vi "subvi_crenelation_reader.vi"(8 "Current Angles":cluster{"Analyser 1":i32, "Analyser 2":i32}, 9 "file (use dialog) 2":path, 10 "Directions":cluster{"Analyser 1":bool, "Analyser 2":bool}, 11 "Analysers Moving?":T1) -> (0 "New Current Angles":cluster{"Analyser 1":i32, "Analyser 2":i32}, 1 "Crenelation \nInterrupts":bool[](array[boolean]) caption="Crenelation Indicators", 3 "Analysers Moving? Output":T1)   [LabVIEW 2014]
doc: "Reads crenelation interrupt (Port 1.1 for analyser 1 and Port 1.5 for analyser 2) states and increments the current angle by 5 degrees if an interrupt fires and appends the new angle to a file specified."
uses:
  Bool Crossing/typedef_twice_bool_crossing.ctl
panel:
  # "INPUTS"
  # "OUTPUTS"
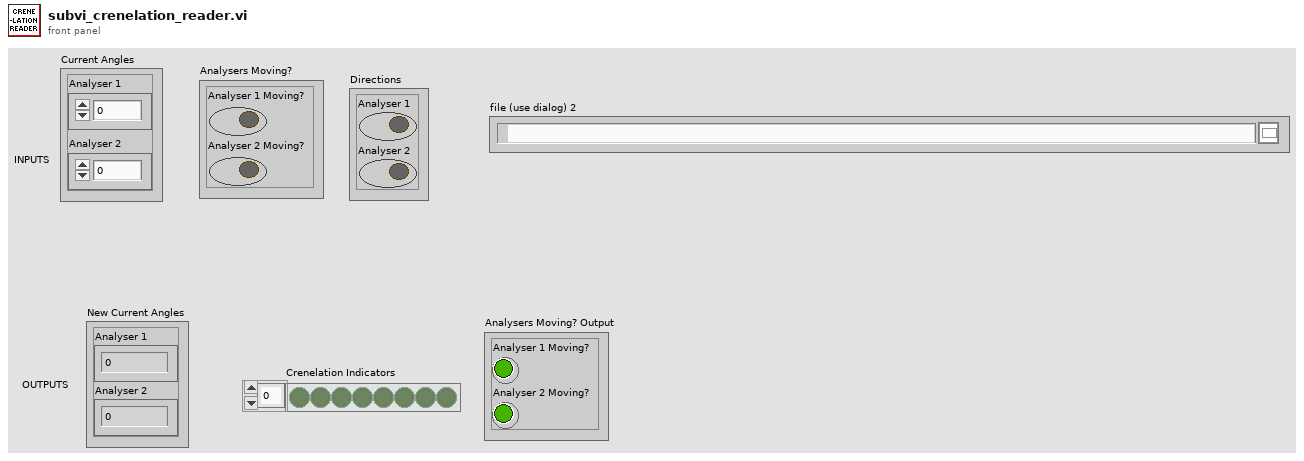
[diagram p1: front panel]
types:
  T1 = cluster{"Analyser 1 Moving?":bool, "Analyser 2 Moving?":bool}
  T2 = typedef "typedef_twice_bool_crossing.ctl" = enum16{"F->T->F", "T->F->T", "Initialise"}
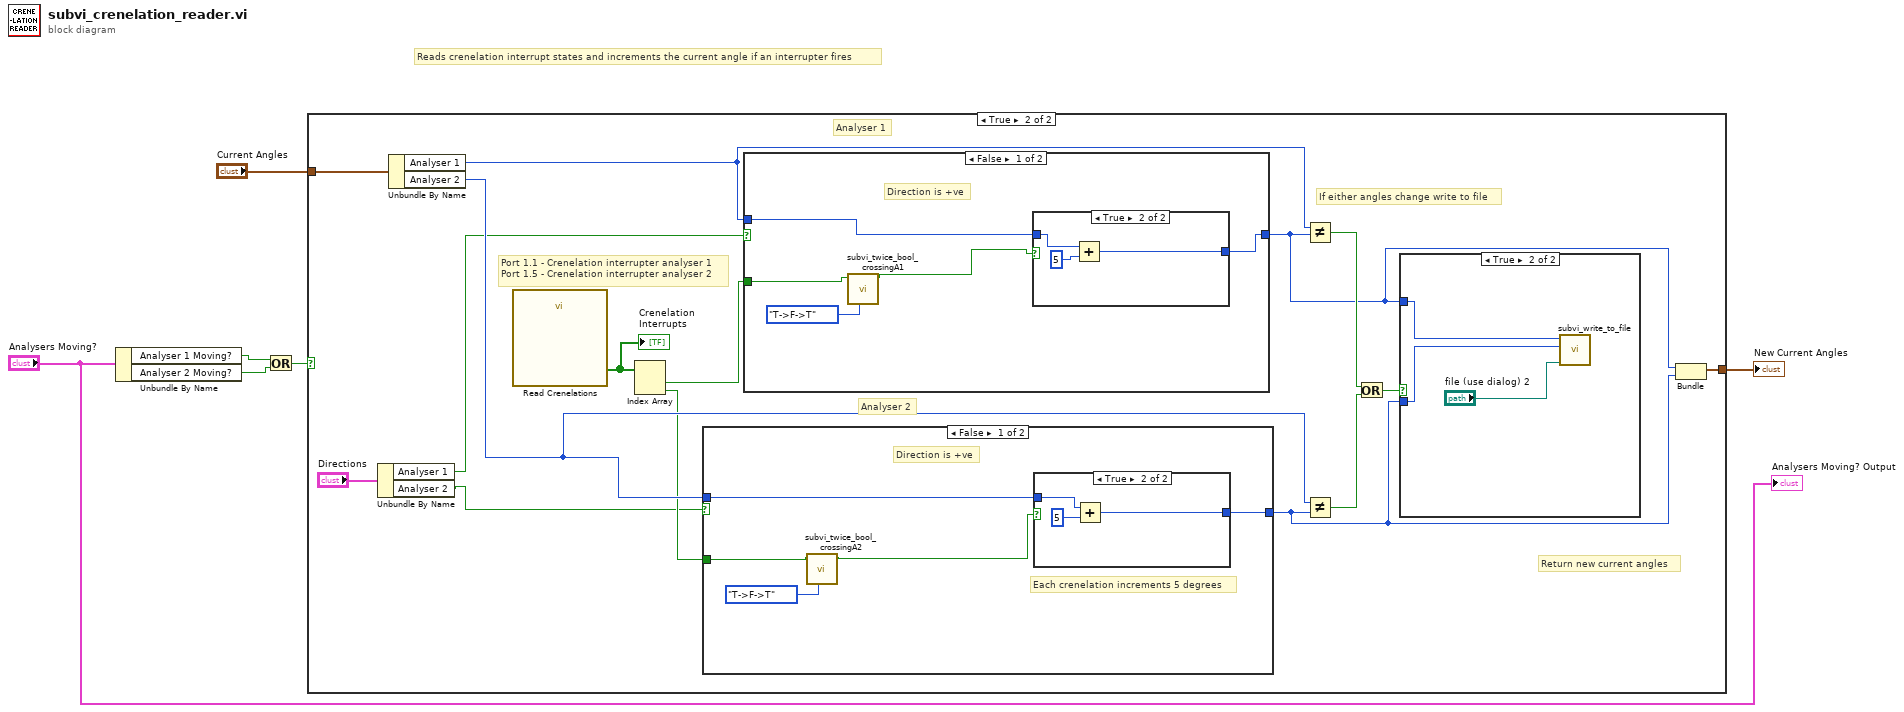
[diagram p0: block diagram]
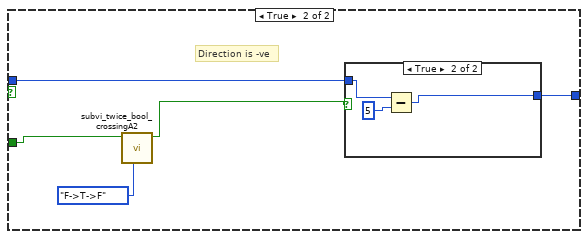
[diagram p4: hidden frame]
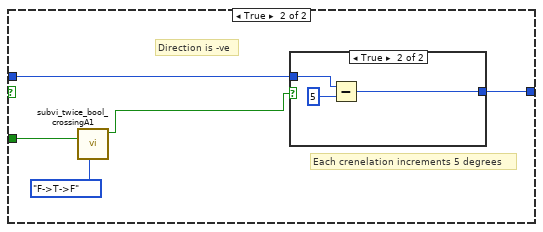
[diagram p8: hidden frame]
diagram:
  # "Reads crenelation interrupt states and increments the current angle if an interrupter fires"
  n1 = Unbundle By Name("Analysers Moving?") -> ("Analyser 1 Moving?"=w5:bool, "Analyser 2 Moving?"=w4:bool)
  n2 = Or(x=w5, y=w4) -> (x .or. y?=w3:bool)
  n3 = case shown="True" w3 {
    tunnel: [w7 w8] -> w2
    tunnel: "Current Angles" -> [w7 w9]
    frame False {
    }
    frame True {
      # "Analyser 2"
      # "Return new current angles"
      # "If either angles change write to file"
      # "Analyser 1"
      # "Port 1.1 - Crenelation interrupter analyser 1\nPort 1.5 - Crenelation interrupter analyser 2"
      n4 = Unbundle By Name("Directions") -> ("Analyser 1"=w12:bool, "Analyser 2"=w11:bool)
      n5 = Unbundle By Name(w9) -> ("Analyser 1"=w19:i32, "Analyser 2"=w18:i32)
      n6 = call "Read Crenelations"() -> ("data"=w15:bool[])  [unwired: 17 in, 2 out]
      "Crenelation \nInterrupts" <- w15
      n7 = Index Array(array=w15) -> (element #1=w14:bool, element #2=w13:bool)  [unwired: 2 in]
      n8 = case shown="False" w11 {
        tunnel: w13 -> [w25 w34]
        tunnel: w18 -> [w27 w36]
        tunnel: [w26 w35] -> w16
        frame False {
          # "Each crenelation increments 5 degrees"
          # "Direction is +ve"
          n9 = call "subvi_twice_bool_crossingA2.vi"("Action"=typedef_twice_bool_crossing."T->F->T", "Input Bool"=w25) -> ("Action Met?"=w24:bool)  [unwired: 8 in, 1 out]
          n10 = case shown="True" w24 {
            tunnel: w27 -> [w28 w31]
            tunnel: [w28 w29] -> w26
            frame False {
            }
            frame True {
              n11 = Add(x=w31, y=5) -> (x+y=w29:i32)
            }
          }
        }
        frame True {
          # "Direction is -ve"
          n12 = call "subvi_twice_bool_crossingA2.vi"("Action"=typedef_twice_bool_crossing."F->T->F", "Input Bool"=w34) -> ("Action Met?"=w33:bool)  [unwired: 8 in, 1 out]
          n13 = case shown="True" w33 {
            tunnel: w36 -> [w37 w40]
            tunnel: [w37 w38] -> w35
            frame False {
            }
            frame True {
              n14 = Subtract(x=w40, y=5) -> (x-y=w38:i32)
            }
          }
        }
      }
      n15 = case shown="False" w12 {
        tunnel: w14 -> [w46 w55]
        tunnel: w19 -> [w48 w57]
        tunnel: [w47 w56] -> w17
        frame False {
          # "Direction is +ve"
          n16 = call "subvi_twice_bool_crossingA1.vi"("Action"=typedef_twice_bool_crossing."T->F->T", "Input Bool"=w46) -> ("Action Met?"=w45:bool)  [unwired: 8 in, 1 out]
          n17 = case shown="True" w45 {
            tunnel: w48 -> [w49 w52]
            tunnel: [w49 w50] -> w47
            frame False {
            }
            frame True {
              n18 = Add(x=w52, y=5) -> (x+y=w50:i32)
            }
          }
        }
        frame True {
          # "Each crenelation increments 5 degrees"
          # "Direction is -ve"
          n19 = call "subvi_twice_bool_crossingA1.vi"("Action"=typedef_twice_bool_crossing."F->T->F", "Input Bool"=w55) -> ("Action Met?"=w54:bool)  [unwired: 8 in, 1 out]
          n20 = case shown="True" w54 {
            tunnel: w57 -> [w58 w61]
            tunnel: [w58 w59] -> w56
            frame False {
            }
            frame True {
              n21 = Subtract(x=w61, y=5) -> (x-y=w59:i32)
            }
          }
        }
      }
      n22 = Not Equal?(x=w19, y=w17) -> (x != y?=w22:bool)
      n23 = Not Equal?(x=w18, y=w16) -> (x != y?=w21:bool)
      n24 = Or(x=w22, y=w21) -> (x .or. y?=w20:bool)
      n25 = case shown="True" w20 {
        tunnel: w17 -> [_ w43]
        tunnel: w16 -> [_ w42]
        frame False {
        }
        frame True {
          n26 = call "subvi_write_to_file.vi"("file (use dialog) in"="file (use dialog) 2", "Analyser2"=w42, "Analyser 1"=w43) -> ()  [unwired: 9 in]
        }
      }
      n27 = Bundle("Analyser 1"=w17, "Analyser 2"=w16) -> (w8:cluster{"Analyser 1":i32, "Analyser 2":i32})  [unwired: 1 in]
    }
  }
  "New Current Angles" <- w2
  "Analysers Moving? Output" <- "Analysers Moving?"
